vi "Pre Launch Init.vi"(11 "IViewModel In":refnum<class "IViewModel.lvclass">) -> (0 "error out":errorcluster, 3 "IViewModel Out":refnum<class "IViewModel.lvclass">)   [LabVIEW 2017, in "IViewModel.lvlib" / "IViewModel.lvclass"]
doc: "(<B>Filename</B>: Actor Framework.lvlib:Actor.lvclass:Pre Launch Init.vi)\n\nDefines behavior that occurs after the Launch Nested Actor method is invoked but before the actor's Actor Core method begins running.\n\nBy default, this method does nothing. A descendant class may override it to define behavior.\n\n<License>\nCopyright © 2017 Composed Systems, LLC | All rights reserved\nwww.composed.io\n\nAuthor: Ethan Stern <ethan.stern@composed.io>\n\nThis software is provided \"AS IS\" WITHOUT WARRANTIES, either express or implied, AND IS FOR EDUCATIONAL PURPOSES ONLY.\n</License>"
uses:
  IViewModel.lvclass
  C:/Program Files (x86)/National Instruments/LabVIEW 2017/vi.lib/ActorFramework/Actor/Actor.lvclass
  C:/Git/mva-framework/Framework/IViewable/IViewable/IViewable.lvclass
  <vilib>/ActorFramework/Actor/Actor.lvclass/Actor.ctl
  <vilib>/ActorFramework/Message Enqueuer/Message Enqueuer.lvclass/Message Enqueuer.ctl
  <vilib>/ActorFramework/Message Enqueuer/Message Priority.ctl
  IViewModel.lvclass/IViewModel.ctl
  IViewable/IViewable/IViewable.lvclass/IViewable.ctl
  <vilib>/ActorFramework/Message Enqueuer/Init from Existing Queue.vi
  <vilib>/ActorFramework/Message Enqueuer/Enqueue.vi
  IViewModel Messages/Launch Root Model Msg/Launch Root Model Msg.lvclass
  C:/Program Files (x86)/National Instruments/LabVIEW 2017/vi.lib/ActorFramework/Message/Message.lvclass
  <vilib>/ActorFramework/Message Priority Queue/Priority Enqueue.vi
  <vilib>/ActorFramework/Message Enqueuer/Message Enqueuer.lvclass
  IViewManager/IViewManager/IViewManager.lvclass
  <vilib>/ActorFramework/Actor/Actor.lvclass
  IViewable/IViewable/IViewable.lvclass
  IViewable/ApplicationStyleReference/ApplicationStyleReference.lvclass
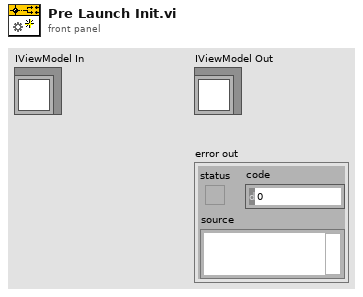
[diagram p1: front panel]
types:
  T1 = typedef "Actor Framework.lvlib/Message Enqueuer.lvclass/Message Priority.ctl" = enum16{"Low", "Normal", "High"}
  T2 = typedef "IViewable.lvlib/ApplicationStyleReference.lvclass/Application Style Reference.ctl" = refnum<data-value>
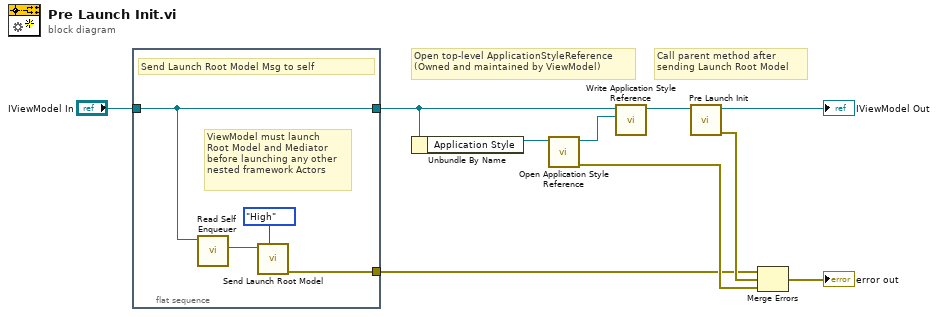
[diagram p0: block diagram]
diagram:
  # "Call parent method after\nsending Launch Root Model"
  # "Open top-level ApplicationStyleReference\n(Owned and maintained by ViewModel)"
  n1 = flat-sequence {
    tunnel: [w13] -> w1
    tunnel: "IViewModel In" -> [w11]
    tunnel: [w11] -> w3
    frame #0 {
      # "ViewModel must launch\nRoot Model and Mediator\nbefore launching any other\nnested framework Actors"
      # "Send Launch Root Model Msg to self"
      n2 = call <vilib>:"Read Self Enqueuer.vi"("Actor"=w11) -> ("Self Enqueuer"=w14:refnum<class "Message Enqueuer.lvclass">)  [unwired: 10 in]
      n3 = call "Send Launch Root Model.vi"("Message Priority (Normal)"=Message_Priority."High", "Message Enqueuer"=w14) -> ("error out"=w13:errorcluster)  [unwired: 8 in, 1 out]
    }
  }
  n4 = Unbundle By Name(w3) -> ("Application Style"=w9:refnum<class "IApplicationStyle.lvclass">)
  n5 = call "Open Application Style Reference.vi"("ApplicationStyle"=w9) -> ("error out"=w6:errorcluster, "Application Style Reference"=w8:T2)  [unwired: 9 in]
  n6 = call "Write Application Style Reference.vi"("Application Style Reference"=w8, "IViewable in"=w3) -> ("IViewable out"=w10:refnum<class "IViewModel.lvclass">)  [unwired: 9 in]
  n7 = call-parent "Pre Launch Init.vi"("IViewManager in"=w10) -> ("error out"=w2:errorcluster, "IViewManager out"=→"IViewModel Out":refnum<class "IViewModel.lvclass">)  [unwired: 9 in]
  n8 = Merge Errors(w1, w2, w6) -> (→"error out":errorcluster)
